vi "Actor Core.vi"(8 "error in":errorcluster, 11 "Pulse Recorder in":refnum<class "NI-Scope Lock-in.lvclass">) -> (0 "error out":errorcluster, 3 "Actor out":refnum<class "Actor.lvclass">)   [LabVIEW 2016, in "NI-Scope Lock-in.lvclass"]
doc: "(<B>Filename</B>: Actor Framework.lvlib:Actor.lvclass:Actor Core.vi)\n\nReceives messages to the actor, reacts to them, and initiates any error handling that may shut the actor down.\n\nDescendant classes may override this VI to append parallel tasks for the actor to complete while it handles messages. Overrides use the Call Parent Method node."
uses:
  NI-Scope Lock-in.lvclass
  <vilib>/ActorFramework/Actor/Actor.lvclass
  NHMFL_Core/Libraries/NI-DAQ/NI-Scope Lock-in Driver/NI-Scope Lock-in Configuration.ctl
  Pulse Recorders/Pulse Recorder/Pulse Recorder.lvclass
panel:
  out "Armed":bool
  out "Name":string
  in  "Configuration":T1={"Points per sine wave"=0, "Rate"=1000000.0, "Re-name channels"=[], "Active channels"="0:1", "Ranges"=[10.0]} {"Ranges" format="%#_6pV"; "Rate" format="%#_8pHz"}
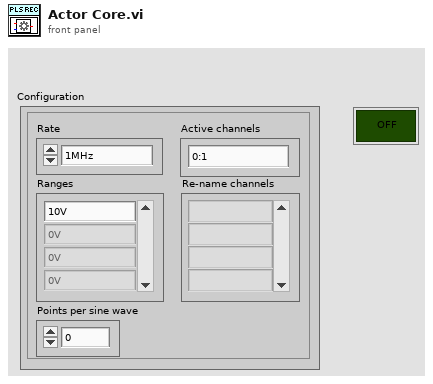
[diagram p1: front panel]
types:
  T1 = typedef "NI-Scope Lock-in Configuration.ctl" = cluster{"Points per sine wave":i32, "Rate":dbl, "Re-name channels":string[], "Active channels":string, "Ranges":dbl[]}
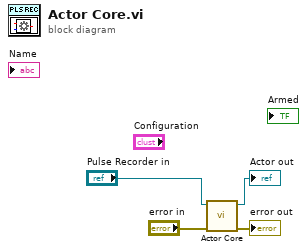
[diagram p0: block diagram]
diagram:
  n1 = call-parent "Actor Core.vi"("error in"="error in", "Pulse Recorder in"="Pulse Recorder in") -> ("error out"=→"error out":errorcluster, "Actor out"=→"Actor out":refnum<class "Actor.lvclass">)  [unwired: 8 in]
